vi "Check & Reset Timestamp.vi"(8 "error in (no error)":errorcluster, 11 "FPGA Ref in":refnum<k20>) -> (0 "error out":errorcluster, 3 "FPGA Ref out":refnum<k20>)   [LabVIEW 2025]
uses:
  <vilib>/rvi/interface/nirviReadWriteControl/nirviReadWriteControl.xnode
  NiFpgaLv.dll
  <vilib>/Utility/error.llb/Error Cluster From Error Code.vi
  <vilib>/rvi/interface/Simulation/niFpgaSimulationCallBeginRW.vi
  <vilib>/rvi/errors/niLvFpgaAdjustHostInterfaceError.vi
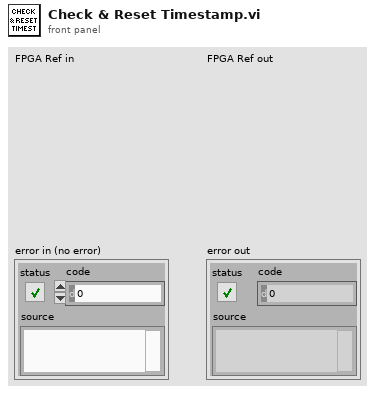
[diagram p1: front panel]
types:
  T1 = enum8{"Idle", "Ready For Start Trigger", "Acquire", "Error"}
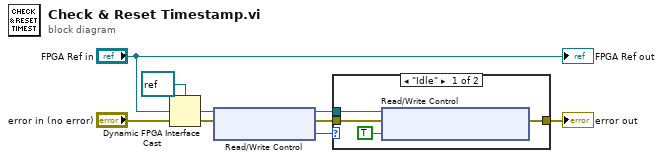
[diagram p0: block diagram]
diagram:
  n1 = Dynamic FPGA Interface Cast(Session In=refnum<k20> refnum ("FPGA VI Reference Out"), Type="FPGA Ref in") -> (Session Out=w6:refnum<k20>)
  n2 = xnode "Read/Write Control"("FPGA VI Reference In"=w6, "error in"="error in (no error)") -> ("FPGA VI Reference Out"=w1:refnum<k20>, "error out"=w3:errorcluster, "global acq state"=w2:T1)
  n3 = case shown="\"Idle\"" w2 {
    tunnel: [w12 w13] -> w4
    tunnel: w3 -> [w11 w13]
    tunnel: w1 -> [w10 _]
    frame "Idle" {
      n4 = xnode "Read/Write Control"("FPGA VI Reference In"=w10, "error in"=w11, "reset timestamp (strobe)"=TRUE) -> ("error out"=w12:errorcluster)  [unwired: 1 out]
    }
    frame Default {
    }
  }
  "error out" <- w4
  "FPGA Ref out" <- "FPGA Ref in"
